vi "ZMQ Req Test.vi"() -> ()   [LabVIEW 2016, in "RemoteControl.ZMQ.lvclass"]
uses:
  RemoteControl.ZMQ.lvclass
panel:
  out "Command Sent":string
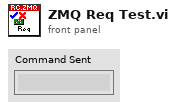
[diagram p1: front panel]
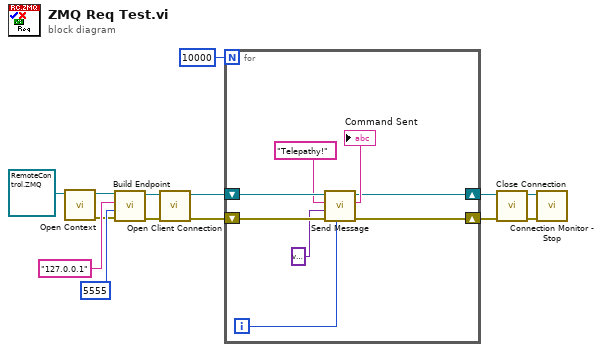
[diagram p0: block diagram]
diagram:
  n1 = call-dynamic "Open Context.vi"("RemoteControl.ZMQ in"=refnum<class "RemoteControl.ZMQ.lvclass"> refnum) -> ("error out"=w4:errorcluster, "RemoteControl.ZMQ out"=w13:refnum<class "RemoteControl.ZMQ.lvclass">)  [unwired: 9 in]
  n2 = call-dynamic "Build Endpoint.vi"("error in (no error)"=w4, "Port"=u16 5555, "Address"="127.0.0.1", "RemoteControl.ZMQ in"=w13) -> ("error out"=w9:errorcluster, "RemoteControl.ZMQ out"=w10:refnum<class "RemoteControl.ZMQ.lvclass">)  [unwired: 6 in]
  n3 = call-dynamic "Open Client Connection.vi"("error in (no error)"=w9, "RemoteControl.ZMQ in"=w10) -> ("error out"=w7:errorcluster, "RemoteControl.ZMQ out"=w8:refnum<class "RemoteControl.ZMQ.lvclass">)  [unwired: 8 in]
  n4 = for {
    N: 10000 -> [_]
    shift-right: [w17] -> w3
    shift-left: w8 -> [w22]
    shift-right: [w16] -> w2
    shift-left: w7 -> [w21]
    i -> [w15]
    n5 = call-dynamic "Send Message.vi"("Message ID"=w15, "error in (no error)"=w21, "Data"=variant, "Command"="Telepathy!", "RemoteControl.ZMQ in"=w22) -> ("error out"=w16:errorcluster, "ACK"=→"Command Sent":string, "RemoteControl.ZMQ out"=w17:refnum<class "RemoteControl.ZMQ.lvclass">)  [unwired: 4 in]
  }
  n6 = call-dynamic "Close Connection.vi"("error in (no error)"=w2, "RemoteControl.ZMQ in"=w3) -> ("error out"=w5:errorcluster, "RemoteControl.ZMQ out"=w6:refnum<class "RemoteControl.ZMQ.lvclass">)  [unwired: 8 in]
  n7 = call-dynamic "Connection Monitor - Stop.vi"("error in (no error)"=w5, "RemoteControl.ZMQ in"=w6) -> ()  [unwired: 8 in, 2 out]
